vi "IMAQ FPGA Camera Link Data to Pixels 1 Tap 24-Bit RGB.vi"(1 "Camera Link Data":cluster{"Port A":u8, "Port B":u8, "Port C":u8}) -> (0 "Pixel":u32)   [LabVIEW 2020]
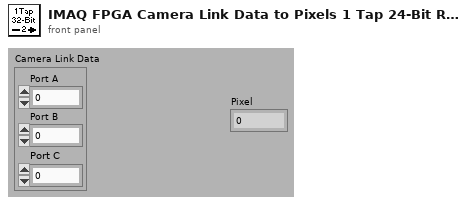
[diagram p1: front panel]
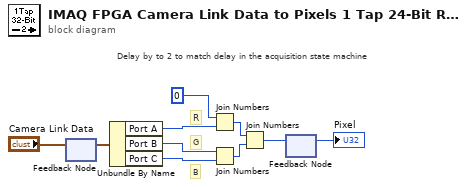
[diagram p0: block diagram]
diagram:
  # "Delay by to 2 to match delay in the acquisition state machine"
  # "B"
  # "G"
  # "R"
  n1 = feedback #1() -> (w5:cluster{"Port A":u8, "Port B":u8, "Port C":u8})  [unwired: 1 in]
  n2 = feedback-in #1("Camera Link Data") -> ()
  n3 = Unbundle By Name(w5) -> ("Port A"=w4:u8, "Port B"=w3:u8, "Port C"=w2:u8)
  n4 = Join Numbers(hi=u8 0, lo=w4) -> ((hi.lo)=w8:u16)
  n5 = Join Numbers(hi=w3, lo=w2) -> ((hi.lo)=w9:u16)
  n6 = Join Numbers(hi=w8, lo=w9) -> ((hi.lo)=w7:u32)
  n7 = feedback-in #2(w7) -> ()
  n8 = feedback #2() -> (→"Pixel":u32)  [unwired: 1 in]
